vi "SteeringControl.vi"(0 "Position (Counts)":i32, 1 "Cluster":cluster{dbl, dbl, dbl}, 3 "Limit":i8, 4 "P_o gain":dbl, 5 "I_o gain":dbl, 6 "error in (no error)":errorcluster, 7 "D_o gain":dbl, 8 "Velocity (Counts/interval)":i32, 9 "P_i gain":dbl, 11 "I_i gain":dbl, 13 "D_i gain":dbl, 15 "Inner PID T/F":bool, 17 "Old (F), new (T) PID":bool) -> (20 "error out":errorcluster, 21 "PWM Out":dbl)   [LabVIEW 2019]
uses:
  <vilib>/myRIO/Instrument Drivers/Onboard IO/PWM/typedefs/PWM Configuration.ctl
  <vilib>/myRIO/Instrument Drivers/Onboard IO/PWM/PWM.lvlib
  <vilib>/myRIO/Common/Instrument Driver Framework/myRIO v1.0/PWM/typedefs/PWM Channels Enum.ctl
  <vilib>/myRIO/Common/Instrument Driver Framework/Utilities/typedefs/Generic FPGA Reference.ctl
  <vilib>/myRIO/Common/Instrument Driver Framework/Utilities/typedefs/myRIO v1.0 Reference.ctl
  <vilib>/myRIO/Common/Instrument Driver Framework/Utilities/typedefs/Hardware Version Enum.ctl
  <vilib>/myRIO/Common/Instrument Driver Framework/Utilities/typedefs/myRIO Generic Hardware Reference.ctl
  <vilib>/myRIO/Instrument Drivers/Onboard IO/PWM/typedefs/PWM Reference.ctl
  <vilib>/myRIO/Instrument Drivers/Onboard IO/PWM/vis/Set Duty Cycle and Frequency.vi
  <vilib>/myRIO/Instrument Drivers/Onboard IO/PWM/vis/myRIO PWM Open.xnode
  <vilib>/myRIO/Common/Instrument Driver Framework/Utilities/vis/Is FPGA Ref Available.vi
  <vilib>/myRIO/Express VI/Onboard IO/PWM/PWM Express VI.xnode
  balancing_dll/Debug/balancing.dll
  <vilib>/myRIO/Common/Instrument Driver Framework/myRIO v1.0/PWM/vis/myRIO v1.1 Open PWM.vi
  <vilib>/userDefined/High Color/nirio_resource_hc.ctl
panel:
  out "Numeric out":dbl
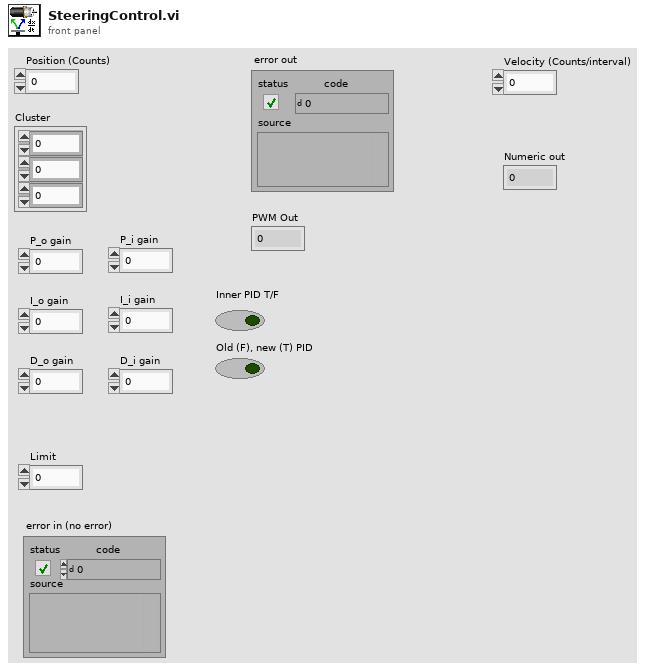
[diagram p1: front panel]
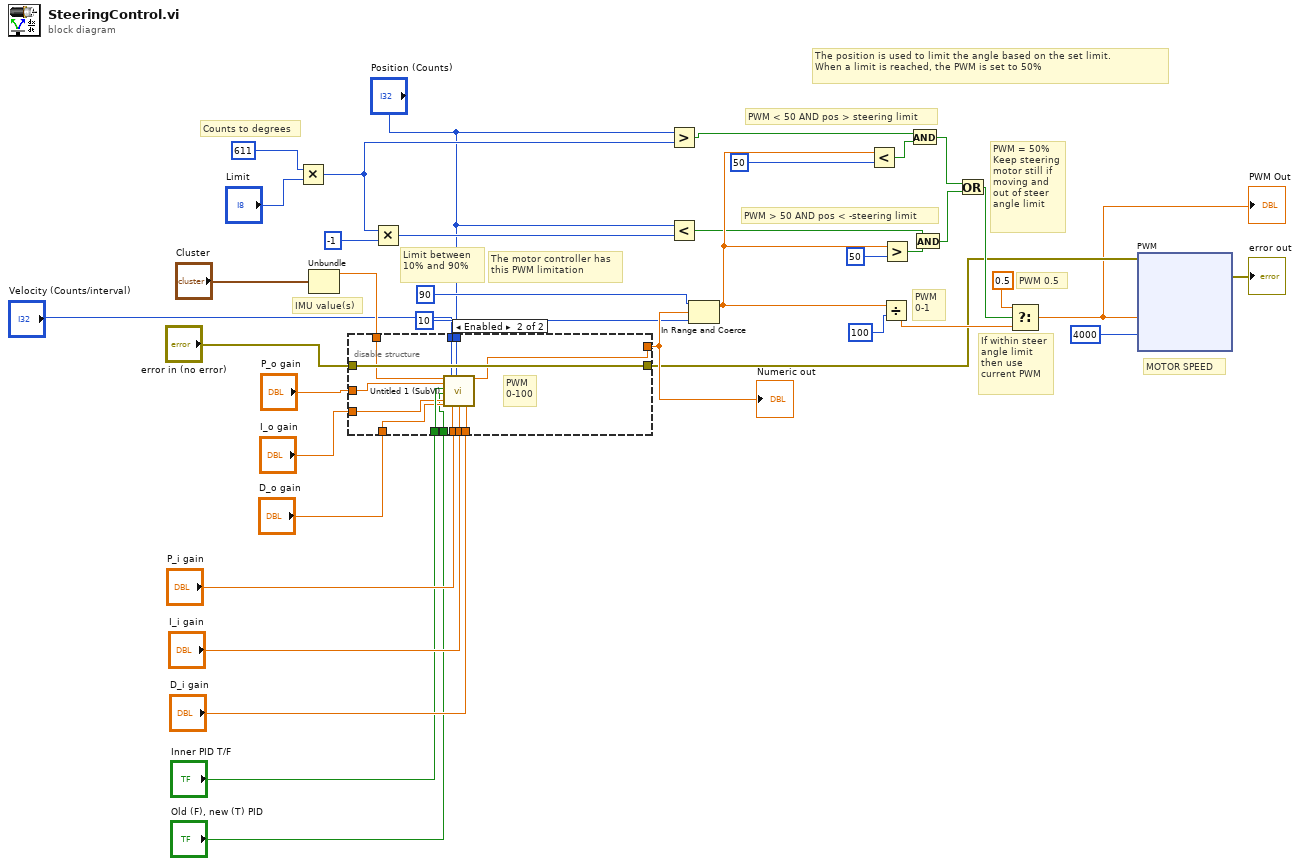
[diagram p0: block diagram]
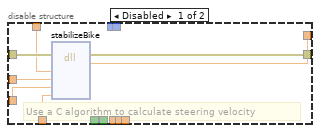
[diagram p2: hidden frame]
diagram:
  # "MOTOR SPEED"
  # "Counts to degrees"
  # "IMU value(s)"
  # "If within steer\nangle limit \nthen use\ncurrent PWM"
  # "PWM 0.5"
  # "PWM = 50%\nKeep steering\nmotor still if\nmoving and\nout of steer\nangle limit"
  # "PWM < 50 AND pos > steering limit"
  # "PWM > 50 AND pos < -steering limit"
  # "PWM\n0-1"
  # "The motor controller has\nthis PWM limitation"
  # "Limit between\n10% and 90%"
  # "The position is used to limit the angle based on the set limit.\nWhen a limit is reached, the PWM is set to 50%"
  n1 = Multiply(x=611, y="Limit") -> (x*y=w14:i32)
  n2 = Unbundle("Cluster") -> (w9:dbl)  [unwired: 2 out]
  n3 = disable-structure shown="Enabled" {
    disable-tunnel: [w45 w57] -> w24
    disable-tunnel: "P_o gain" -> [w44 w51]
    disable-tunnel: "I_o gain" -> [w43 w50]
    disable-tunnel: "error in (no error)" -> [w41 w58]
    disable-tunnel: [w40 w58] -> w11
    disable-tunnel: w9 -> [w39 w52]
    disable-tunnel: "P_i gain" -> [_ w56]
    disable-tunnel: "I_i gain" -> [_ w55]
    disable-tunnel: "D_i gain" -> [_ w54]
    disable-tunnel: "D_o gain" -> [w42 w49]
    disable-tunnel: "Inner PID T/F" -> [_ w53]
    disable-tunnel: "Old (F), new (T) PID" -> [_ w48]
    disable-tunnel: "Velocity (Counts/interval)" -> [_ w47]
    disable-tunnel: "Position (Counts)" -> [_ w46]
    frame Disabled {
      # "Use a C algorithm to calculate steering velocity"
      n4 = dll-call lib="C:/Users/AutoBike22 - Layos/Documents/LabVIEWorkspace/balancing_dll/Debug/balancing.dll" fn="stabilizeBike"(error in=w41, "rollRate"=w39, "Kp"=w44, "Ki"=w43, "Kd"=w42) -> (error out=w40:errorcluster, "return type"=w45:dbl)  [unwired: 6 in, 1 out]
    }
    frame Enabled {
      # "PWM\n0-100"
      n5 = call "Untitled 1 (SubVI).vi"("Numeric in"=w52, "P_outer gain"=w51, "Inner PID T/F"=w53, "Old (F), new (T) PID"=w48, "I_outer gain"=w50, "D_outer gain"=w49, "Velocity (Counts/interval)"=w47, "P_inner gain"=w56, "Position (Counts)"=w46, "I_inner gain"=w55, "D_inner gain"=w54) -> ("Numeric out"=w57:dbl)  [unwired: 8 in]
    }
  }
  "Numeric out" <- w24
  n6 = Multiply(x=w14, y=-1) -> (x*y=w16:i32)
  n7 = Greater?(x="Position (Counts)", y=w14) -> (0:w38:bool)
  n8 = Less?(x="Position (Counts)", y=w16) -> (x < y?=w26:bool)
  n9 = In Range and Coerce(upper limit=90, x=w24, lower limit=10) -> (coerced(x)=w30:dbl)  [unwired: 1 out]
  n10 = Less?(x=w30, y=50) -> (x < y?=w29:bool)
  n11 = Divide(x=w30, y=100) -> (x/y=w35:dbl)
  n12 = Greater?(x=w30, y=50) -> (0:w27:bool)
  n13 = And(x=w38, y=w29) -> (x .and. y?=w32:bool)
  n14 = And(x=w26, y=w27) -> (x .and. y?=w33:bool)
  n15 = Or(x=w32, y=w33) -> (x .or. y?=w34:bool)
  n16 = Select(t=0.5, s=w34, f=w35) -> (s? t:f=w10:dbl)
  "PWM Out" <- w10
  n17 = xnode "PWM"("Duty Cycle"=w10, "Frequency [Hz]"=4000, "error in (no error)"=w11) -> ("error out"=→"error out":errorcluster)
